vi "Scan Setup.vi"(8 "error in (no error)":errorcluster, 11 "Pulse Gen Scan in":refnum<class "Pulse Gen Scan.lvclass">) -> (0 "error out":errorcluster, 3 "Pulse Gen Scan out":refnum<class "Pulse Gen Scan.lvclass">)   [LabVIEW 2009, in "Pulse Gen Scan.lvclass"]
uses:
  Pulse Gen Scan.lvclass
  Scanner/Scanner.lvclass
  Global/GPIB Numbers.vi
  Pulse Gen Scan.lvclass/Pulse Gen Scan.ctl
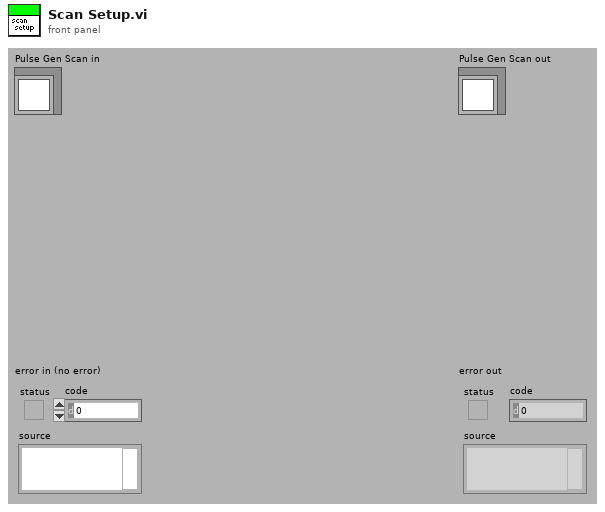
[diagram p1: front panel]
types:
  T1 = typedef "GPIB Type Def.ctl" = cluster{"Name":string, "bus":dbl, "GPIB":dbl, "GPIB as string":string, "byte":i32, "VISA Resource Name":refnum<visa-resource-name>}
  T2 = enum16{"Internal Oscillator", "Internal PLL", "Clock Input"}
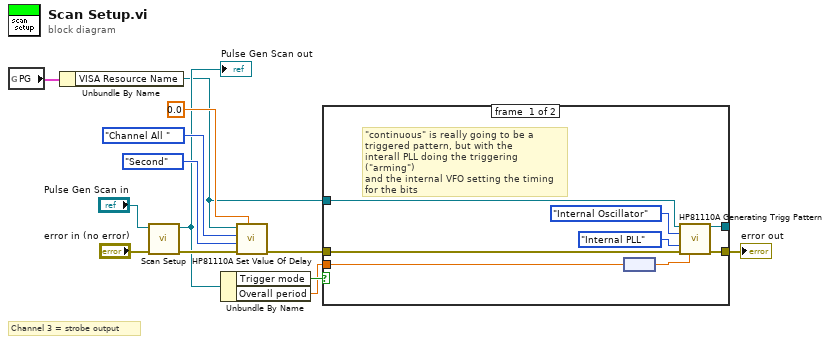
[diagram p0: block diagram]
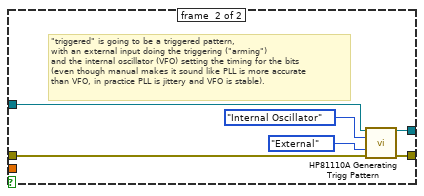
[diagram p2: hidden frame]
diagram:
  # "Channel 3 = strobe output"
  n1 = global read "GPIB Numbers.vi" "PG"() -> (w11:T1)
  n2 = Unbundle By Name(w11) -> ("VISA Resource Name"=w3:refnum<visa-resource-name>)
  n3 = call-parent "Scan Setup.vi"("error in (no error)"="error in (no error)", "Scanner in"="Pulse Gen Scan in") -> ("error out"=w7:errorcluster, "Scanner out"=w6:refnum<class "Pulse Gen Scan.lvclass">)  [unwired: 8 out]
  "Pulse Gen Scan out" <- w6
  n4 = Unbundle By Name(w6) -> ("Trigger mode"=w5:bool, "Overall period"=w4:dbl[unit])
  n5 = call "HP81110A Set Value Of Delay.vi"("Delay Value (0.0)"=0.0, "error in (no error)"=w7, "Delay Unit (0:Second)"=enum16{"Second", "Percent", "Degree", "Radians"}."Second", "Channel (1:Channel 1)"=enum16{"Channel All ", "Channel 1", "Channel 2"}."Channel All ", "VISA session"=w3) -> ("error out"=w2:errorcluster)  [unwired: 6 out]
  n6 = case shown="True" w5 {
    tunnel: w2 -> [w18 w25]
    tunnel: [w17 w24] -> w1
    tunnel: w3 -> [w19 w26]
    tunnel: w4 -> [w16 _]
    tunnel: [w14 w22] -> _
    frame #0 {
      # "\"continuous\" is really going to be a \ntriggered pattern, but with the \ninterall PLL doing the triggering (\"arming\")\nand the internal VFO setting the timing \nfor the bits"
      n7 = node(w16) -> (w15:dbl)
      n8 = call "HP81110A Generating Trigg Pattern.vi"("VISA session"=w19, "Period Source (0:Internal Oscillator)"=T2."Internal Oscillator", "Trigger Source (0:Internal PLL)"=enum16{"Internal PLL", "External", "Manual"}."Internal PLL", "error in (no error)"=w18, "PLL Value (10.0E-6)"=w15) -> ("dup VISA session"=w14:refnum<visa-resource-name>, "error out"=w17:errorcluster)  [unwired: 3 in, 6 out]
    }
    frame #1 {
      # "\"triggered\" is going to be a triggered pattern, \nwith an external input doing the triggering (\"arming\")\nand the internal oscillator (VFO) setting the timing for the bits \n(even though manual makes it sound like PLL is more accurate \nthan VFO, in practice PLL is jittery and VFO is stable)."
      n9 = call "HP81110A Generating Trigg Pattern.vi"("VISA session"=w26, "Period Source (0:Internal Oscillator)"=T2."Internal Oscillator", "Trigger Source (0:Internal PLL)"=enum16{"Internal PLL", "External", "Manual"}."External", "error in (no error)"=w25) -> ("dup VISA session"=w22:refnum<visa-resource-name>, "error out"=w24:errorcluster)  [unwired: 4 in, 6 out]
    }
  }
  "error out" <- w1
